vi "Add Rational Polynomials (DBL).vi"(4 "threshold type":T1 items=["Absolute Value", "Relative Value"], 6 "threshold":dbl, 8 "Denominator 2":dbl[](array[numeric]) format="%#.2g", 9 "Numerator 2":dbl[](array[numeric]) format="%#.2g", 10 "Denominator 1":dbl[](array[numeric]) format="%#.2g", 11 "Numerator 1":dbl[](array[numeric]) format="%#.2g") -> (0 "error":i32, 2 "Denominator Out":dbl[](array[numeric]) format="%#.2g", 3 "Numerator Out":dbl[](array[numeric]) format="%#.2g")   [LabVIEW 2014, in "NI_AALPro.lvlib"]
doc: "Adds the rational polynomials G1 and G2. The data types you wire to the <B>Numerator 1</B>, <B>Denominator 1</B>, <B>Numerator 2</B>, and <B>Denominator 2</B> inputs determine the polymorphic instance to use."
uses:
  NI_AALPro.lvlib
  Remove Zero Threshold Type.ctl
  Multiply Polynomials (DBL).vi
  Add Polynomials (DBL).vi
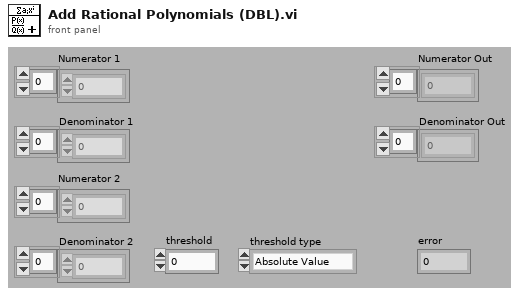
[diagram p1: front panel]
types:
  T1 = typedef "NI_AALPro.lvlib/Remove Zero Threshold Type.ctl" = u16
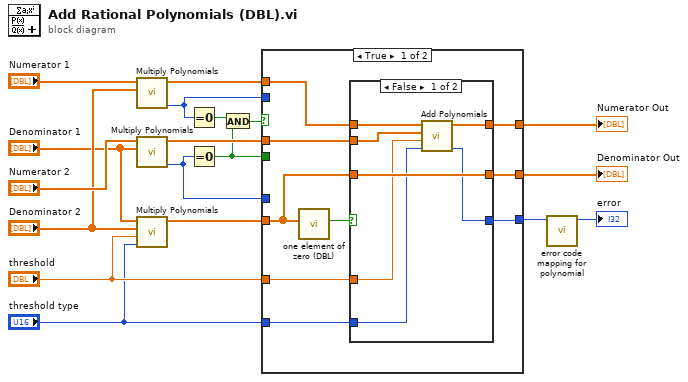
[diagram p0: block diagram]
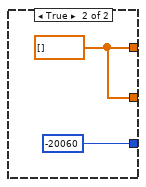
[diagram p2: hidden frame]
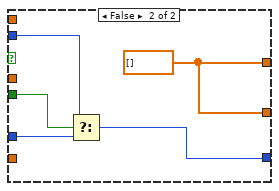
[diagram p3: hidden frame]
diagram:
  n1 = call-poly "Multiply Polynomials.vi"("Q(x)"="Denominator 2", "P(x)"="Numerator 1") -> ("error"=w6:i32, "P(x)*Q(x)"=w4:dbl[])  [unwired: 8 in]
  n2 = call-poly "Multiply Polynomials.vi"("Q(x)"="Denominator 1", "P(x)"="Numerator 2") -> ("error"=w7:i32, "P(x)*Q(x)"=w16:dbl[])  [unwired: 8 in]
  n3 = call-poly "Multiply Polynomials.vi"("threshold type"="threshold type", "threshold"="threshold", "Q(x)"="Denominator 2", "P(x)"="Denominator 1") -> ("P(x)*Q(x)"=w13:dbl[])  [unwired: 6 in, 1 out]
  n4 = Equal To 0?(x=w6) -> (x = 0?=w9:bool)
  n5 = Equal To 0?(x=w7) -> (x = 0?=w8:bool)
  n6 = And(x=w9, y=w8) -> (x .and. y?=w10:bool)
  n7 = case shown="True" w10 {
    tunnel: w4 -> [w27 _]
    tunnel: w16 -> [w26 _]
    tunnel: [w25 w41] -> w15
    tunnel: w13 -> [w23 _]
    tunnel: [w21 w41] -> w14
    tunnel: [w22 w37] -> w12
    tunnel: w8 -> [_ w40]
    tunnel: w7 -> [_ w39]
    tunnel: w6 -> [_ w38]
    tunnel: "threshold" -> [w20 _]
    tunnel: "threshold type" -> [w19 _]
    frame True {
      n8 = call "one element of zero (DBL).vi"("Array in"=w23) -> ("equal [0]?"=w24:bool)  [unwired: 10 in]
      n9 = case shown="False" w24 {
        tunnel: w27 -> [w34 _]
        tunnel: w26 -> [w33 _]
        tunnel: [w32 w36] -> w25
        tunnel: w23 -> [w31 _]
        tunnel: [w30 -20060 ("divide by zero")] -> w22
        tunnel: [w31 w36] -> w21
        tunnel: w20 -> [w29 _]
        tunnel: w19 -> [w28 _]
        frame False {
          n10 = call-poly "Add Polynomials.vi"("threshold type"=w28, "threshold"=w29, "Q(x)"=w33, "P(x)"=w34) -> ("error"=w30:i32, "P(x)+Q(x)"=w32:dbl[])  [unwired: 6 in]
        }
        frame True {
          w36 = dbl[] [] ("BDL")
        }
      }
    }
    frame False {
      w41 = dbl[] [] ("BDL")
      n11 = Select(t=w38, s=w40, f=w39) -> (s? t:f=w37:i32)
    }
  }
  "Numerator Out" <- w15
  "Denominator Out" <- w14
  n12 = call "error code mapping for polynomial.vi"("error in"=w12) -> ("error out"=→"error":i32)  [unwired: 10 in]
